vi "AM Update Low Level.vi"(7 "Control Name":string, 8 "error in (no error)":errorcluster, 10 "Value":variant) -> (0 "error out":errorcluster)   [LabVIEW 2020, in "Test Driver.lvlib"]
uses:
  Test Driver.lvlib
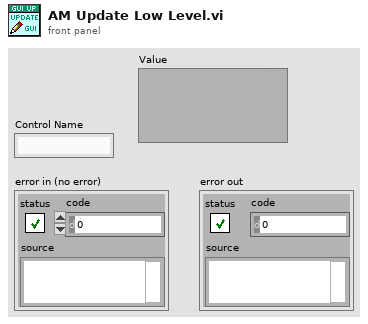
[diagram p1: front panel]
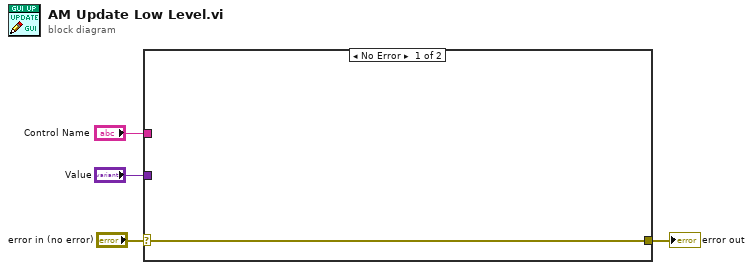
[diagram p0: block diagram]
diagram:
  n1 = case shown="No Error" "error in (no error)" {
    selector: "error in (no error)" -> [w5 w6]
    tunnel: [w5 w6] -> w3
    tunnel: "Control Name" -> [_ _]
    tunnel: "Value" -> [_ _]
    frame No Error {
    }
    frame Error {
    }
  }
  "error out" <- w3
